vi "AcquireData.vi"(8 "error in (no error)":errorcluster, 11 "config in":T1) -> (0 "error out":errorcluster, 3 "config out":T1)   [LabVIEW 2017, in "ScanEngine.lvlib"]
uses:
  <vilib>/addons/InsightCM/Devices/Shared/Common/ScanEngine/ScanEngine.lvlib
  <vilib>/addons/InsightCM/Devices/Shared/Common/ScanEngine/controls/Configuration.ctl
  <vilib>/addons/InsightCM/Devices/Shared/Common/ScanEngine/controls/Group.ctl
  <vilib>/addons/InsightCM/Devices/Shared/Common/ScanEngine/controls/Channel.ctl
  <vilib>/Utility/Data Type/Type Definitions/Data Type.ctl
  <vilib>/addons/InsightCM/MessageBus/Base/controls/KeyValuePair.ctl
  <vilib>/addons/PointValueMap/subVIs/Point_Write_double.vi
  <vilib>/addons/PointValueMap/PointValueMap.lvlib
  <vilib>/Utility/Data Type/NI_Data Type.lvlib
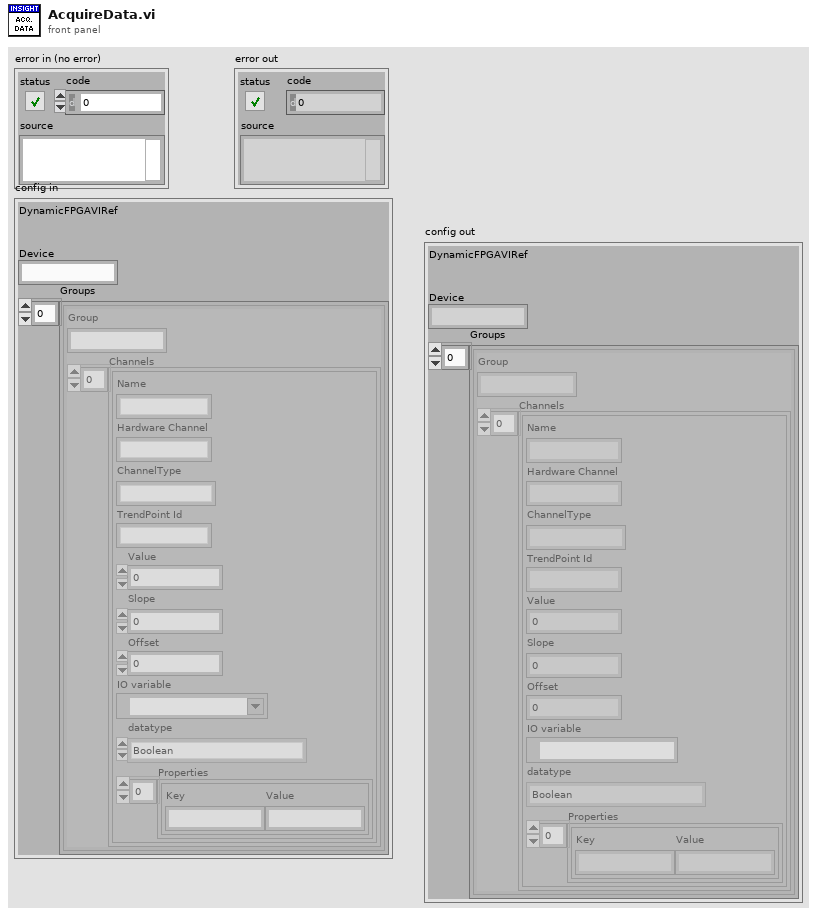
[diagram p1: front panel]
types:
  T1 = typedef "ScanEngine.lvlib/Configuration.ctl" = cluster{"DynamicFPGAVIRef":refnum<k20>, "Device":string, "Groups":T2[]}
  T2 = typedef "ScanEngine.lvlib/Group.ctl" = cluster{"Group":string, "Channels":T3[]}
  T3 = typedef "ScanEngine.lvlib/Channel.ctl" = cluster{"Name":string, "Hardware Channel":string, "ChannelType":string, "TrendPoint Id":string, "Value":sgl, "Slope":dbl, "Offset":dbl, "IO variable":refnum<k21>, "datatype":T4, "Properties":T5[]}
  T4 = typedef "NI_Data Type.lvlib/Data Type.ctl" = enum8{"Invalid Type", "Void", "I8", "I16", "I32", "I64", "U8", "U16", "U32", "U64", "Single Float", "Double Float", "Extended Float", "Single Complex", "Double Complex", "Extended Complex", "Enum U8", "Enum U16", "Enum U32", "Enum U64", "Single Float With Unit", "Double Float With Unit", "Extended Float With Unit", "Single Complex with Unit", "Double Complex with Unit", "Extended Complex with Unit", "Boolean", "String", "Path", "Picture", "Tag", "Array", "Cluster", "Variant", "LV Variant", "Waveform", "Timestamp", "Digital Waveform", "Digital Data", "ExpressData", "Refnum", "External Data", "VI", "Poly VI", "LabVIEW Class Instance", "Fixed Point"}
  T5 = typedef "KeyValuePair.ctl" = cluster{"Key":string, "Value":string}
  T6 = typedef "PointValueMap.lvlib/PointMap.ctl" = refnum<data-value>
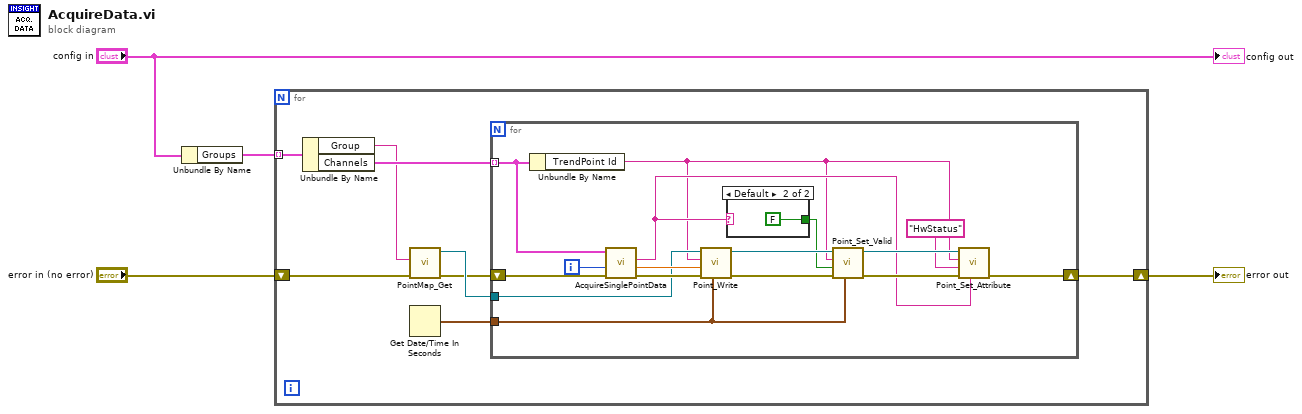
[diagram p0: block diagram]
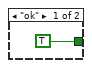
[diagram p2: hidden frame]
diagram:
  n1 = Unbundle By Name("config in") -> ("Groups"=w4:T2[])
  n2 = for {
    shift-right: [w5] -> w2
    shift-left: "error in (no error)" -> [w6]
    tunnel: w4 -> [w11] mode=indexing
    n3 = Unbundle By Name(w11) -> ("Group"=w9:string, "Channels"=w10:T3[])
    n4 = call <vilib>:"PointMap_Get.vi"("error in (no error)"=w6, "Name"=w9) -> ("error out"=w7:errorcluster, "Map Out"=w8:T6)  [unwired: 7 in, 1 out]
    n5 = Get Date/Time In Seconds() -> (seconds since 1Jan1904=w12:timestamp)
    n6 = for {
      shift-right: [w16] -> w5
      shift-left: w7 -> [w28]
      tunnel: w12 -> [w19]
      tunnel: w10 -> [w26] mode=indexing
      tunnel: w8 -> [w23]
      i -> [w27]
      n7 = Unbundle By Name(w26) -> ("TrendPoint Id"=w14:string)
      n8 = call <vilib>:"AcquireSinglePointData.vi"("error in (no error)"=w28, "Numeric"=w27, "Channel"=w26) -> ("error out"=w24:errorcluster, "Value"=w25:dbl, "Status"=w15:string)  [unwired: 6 in]
      n9 = call-poly <vilib>:"Point_Write.vi"("Time Stamp"=w19, "Error In"=w24, "Value"=w25, "Tag"=w14, "Map"=w23) -> ("Error Out"=w21:errorcluster, "Map Out"=w22:T6)  [unwired: 5 in]
      n10 = case shown="Default" w15 {
        tunnel: [TRUE ("Valid?") FALSE ("Valid?")] -> w20
        frame "ok" {
        }
        frame Default {
        }
      }
      n11 = call <vilib>:"Point_Set_Valid.vi"("Timestamp"=w19, "Error In"=w21, "Valid?"=w20, "Tag"=w14, "Map"=w22) -> ("Error Out"=w17:errorcluster, "Map Out"=w18:T6)  [unwired: 5 in]
      n12 = call <vilib>:"Point_Set_Attribute.vi"("Value"=w15, "Error In"=w17, "Attribute"="HwStatus", "Tag"=w14, "Map"=w18) -> ("Error Out"=w16:errorcluster)  [unwired: 5 in, 1 out]
    }
  }
  "error out" <- w2
  "config out" <- "config in"
